vi "Setup 4 Oscilloscope.vi"() -> ()   [LabVIEW 2017]
uses:
  SignalConversion/DAQChannelRawData.ctl
  SignalConversion/ScaledData.ctl
  SignalConversion/Measrured TrapXYZ.ctl
  SignalConversion/Data Before Angle Compensation.ctl
  SignalConversion/Angle compensated data.ctl
  SignalConversion/XYZ Signals.ctl
  SignalConversion/Set TrapXYZ.ctl
  Initialization/New Param_170907.ctl
  Initialization/ManualCtrl.ctl
  Initialization/CylinderCalibrNew.ctl
  SignalConversion/DAQChannelOffsets.ctl
  <vilib>/Analysis/Matrix/Datatypes/RealMatrix.ctl
  <vilib>/Platform/TimedLoop/XDataNode/timing_clust.ctl
  <vilib>/Platform/TimedLoop/XDataNode/nitl_modes.ctl
  <vilib>/Platform/TimedLoop/XDataNode/wakeup.ctl
  <vilib>/Analysis/baseanly.llb/Mean (DBL).vi
  <vilib>/Utility/file.llb/Read Delimited Spreadsheet (DBL).vi
  <vilib>/Utility/file.llb/Write Delimited Spreadsheet (DBL).vi
  <vilib>/platform/TimedLoop/XDataNode/XDataNode.xnode
  Data aquisition/Data aquisition.lvlib
  BasicVIs/BasicVIs.lvlib
  SignalConversion/SignalConverson.lvlib
  <vilib>/Analysis/NI_AALBase.lvlib
  Initialization/FileManagement/FileManagement.lvlib
  <vilib>/Platform/TimedLoop/XDataNode/XDNodeRunTimeDep.lvlib
  Initialization/Initialization.lvlib
  <vilib>/Analysis/Matrix/NI_Matrix.lvlib
panel:
  out "Temperature":string
  out "#Recoreded":i32
  out "Frames":i32
  in  "Oscilloscope sampling Rate":i32=100
  in  "Tab Control":T1(tab)
  out "Temperature":dbl(graph)
  out "Trap height 2":dbl(graph)
  in  "Ignore HF and XYFTC calibration":bool=TRUE
  out "scan backlog:":u32
  out "no error?":bool=TRUE
  out "Torque [pNnm]":dbl(graph)
  out "Trap height":dbl(graph)
  out "Zforce [pN]":dbl(graph)
  out "ellipiticity out":dbl(knob)=10.0 scale=-0.5..0.5
  out "Vy\n            [V]":dbl(knob)=10.0 scale=-0.5..0.5
  out "Vx\n            [V]":dbl(knob)=10.0 scale=-0.5..0.5
  out "Vsum\n            [V]":dbl(knob)=10.0 scale=0.0..10.0
  out "Power meter\n            [mW]":dbl(knob)=500.0 scale=0.0..200.0
  in  "Initialize":bool
  in  "STOP":bool
  in  "Oscilloscope calibration file save path":path=path "V:/Oslo/Setup 4 temp files/Oscilloscope_offset_gain.ini.txt"
  in  "Cal 1":bool
  in  "Cal 2":bool
  in  "Temp file for calibration (channel voltages from control software)":path=path "V:/Oslo/Setup 4 temp files/all channel signals.txt"
  in  "Params measured by control program":path=path "Y:/Setup4/Setup 4 temp files/config of last run.bin"
  in  "Channel gain and offset file (mapping voltages from \"oscilloscope comuputer\" to \"control computer\")":path=path "Y:/Setup4/Setup 4 temp files/Oscilloscope_offset_gain.ini.txt"
  in  "window smooth size (default = 10 points)":i32=10
  in  "Data process in oscilloscope (2,default)":i32(ring)=2 items=["0. Do not compensate, do not calculate polarization angle", "1. Calculate angle, but do not compensate any signal", "2. Compensate all signals by angular gain", "3. Do not scale (show raw voltage signals)"]
  out "point 1 calibration":dbl[][](array[numeric])
  out "Array":T2[](array[typedef])
  out "gains and offsets of all channels":dbl[][](array[numeric])
  in  "Record all channel":bool
  out "error out":errorcluster
  out "Params out":T3={"Manual Control"={"Rotation Control"={"Phase"=0.0, "A amp (0-120)"=75.0, "B amp (0-120)"=53.3, "mean freq  [MHz]\ndefault 39.99"=40.0, "freq difference [Hz]"=2.0, "Enable A"=TRUE, "Enable B"=TRUE}, "X piezo\n [nm]"=nan, "Y peizo\n [nm]"=nan, "-Z piezo\n [nm]"=nan, "AOM0 \nPower"=nan}, "Piezo Calibr"={"Px2Vx(AO)"=nan, "Py2Vy(AO)"=nan, "Pz2Vz(AO)"=nan, "Min Px"=nan, "Min Py"=0.0, "Min Pz"=nan, "Max Px"=nan, "Max Py"=nan, "Max Pz"=nan, "Vx0 (V)"=nan, "Vy0 (V)"=nan, "Vz0 (V)"=nan}, "Instrument Calibr"={"Angular compensation coeffs"=[], "TetherCenter"={"TrapX_AO 0 [nm]"=nan, "TrapY_AO 0 [nm]"=nan, "TrapZ_AO 0 [nm]"=nan}, "XYZsignal baseline"={"Xsignal0"=nan, "Ysignal0"=nan, "Zsignal0"=nan, "Zsig slope"=nan, "Z bead0"=nan}, "S and P to Vs0"={"Vs0/P"=1.0, "Vs0/S"=1.0}, "Psi"=nan, "ePS:eRL drift correlation"={"Interc P"=nan, "Slope P"=nan, "Interc S"=nan, "Slope S"=nan}, "Current piezo volt AO"={"Vpx_AO [V]"=nan, "Vpy_AO [V]"=nan, "Vpz_AO [V]"=nan}}, "Cylinder Calibr"={"ZStiff"=nan, "Zsens"=nan, "AngStiff"=nan, "XStiff"=nan, "Xsens"=nan, "MaxEllip"=nan, "YStiff"=nan, "Ysens"=nan, "FocalShift"=nan, "Sfz"=nan, "1/Sz"=nan, "Stau"=nan, "Sfx"=nan, "1/Sx"=nan, "1/Sang"=nan, "Sfy"=nan, "1/Sy"=nan, "1/focal"=nan}, "DAQParams"={"Buffer size"=0.0, "Scanning rate"=0.0, "Average"=0.0, "Sampling rate"=0.0, "set dt"=0.0}, "DAQ channel offsets"={"A0 [V]"=0.0, "D0 [V]"=0.0, "P0  [V]"=0.0, "S0 [V]"=0.0, "L0 [V]"=0.0, "R0 [V]"=0.0, "Vpx0 [V]"=0.0, "Vpy0 [V]"=0.0, "Vpz0 [V]"=0.0, "Vsum0 [V]"=0.0, "Vpx_AO0 [V]"=0.0, "Vpy_AO0 [V]"=0.0, "Vpz_AO0 [V]"=0.0}, "Z bead polynomial coeffs"=[nan, nan, nan, nan], "Skip button ref"=refnum, "z bead lookup table"={"z signal"=[], "z bead"=[]}, "SP->power Matrix"=[], "Ms2p"=[], "Mp2s"=[], "Polynomial coeff V_px,y,z 2 position (nm)"=[], "task in"=""} {"Instrument Calibr"."Psi" format="%#_2f"; "Manual Control"."Y peizo\n [nm]" scale=0.0..7000.0; "Manual Control"."AOM0 \nPower" scale=0.0..1.0; "Manual Control"."X piezo\n [nm]" scale=0.0..7000.0; "Manual Control"."Rotation Control"."freq difference [Hz]" step=0.5; "Manual Control"."Rotation Control"."mean freq  [MHz]\ndefault 39.99" min=0.0 step=0.01; "Manual Control"."Rotation Control"."B amp (0-120)" min=0.0 max=120.0 step=0.1; "Manual Control"."Rotation Control"."A amp (0-120)" min=0.0 max=120.0 step=0.1; "Manual Control"."Rotation Control"."Phase" scale=0.0..360.0; "Manual Control"."-Z piezo\n [nm]" scale=1000.0..7000.0}
  out "Scaled data":T8
  out "all channels":dbl[][](graph)
  # "Set piezo xy and trap height to zero, turn off AOM A and B, click on \"Setup 4 Control Software: Tools: record all channel raw voltages\""
  # "Set piezo xy and trap height to max, turn on AOM A and B, set  the laser power to max and adjust the phase to achieve A detector voltage = D detector voltage (the 2nd waveform chart, show \"A and D detector [V]\"). Then click on \"Setup 4 Control Software\": tab\" Calibration Tools\" : Bottom \"record all channel raw voltages\""
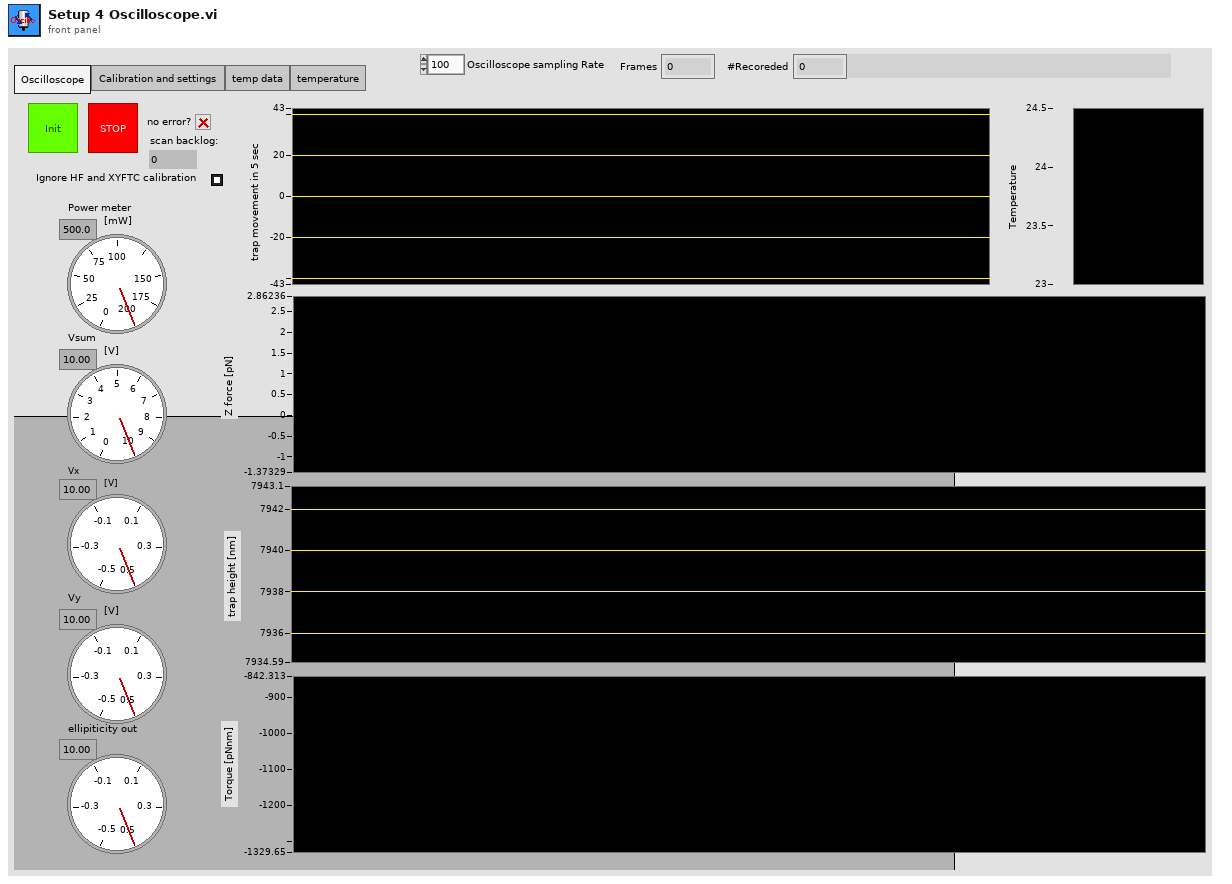
[diagram p1: front panel]
types:
  T1 = enum32{"Oscilloscope", "Calibration and settings ", "temp data", "temperature"}
  T2 = typedef "SignalConverson.lvlib/DAQChannelRawData.ctl" = cluster{"V_A' [V]":dbl, "V_D' [V]":dbl, "V_P'  [V]":dbl, "V_S' [V]":dbl, "V_L' [V]":dbl, "V_R' [V]":dbl, "V_sum' [V]":dbl, "V_x [V]":dbl, "V_y [V]":dbl, "V_px' [V]":dbl, "V_py' [V]":dbl, "V_pz' [V]":dbl, "dt [s]":dbl, "Vpx_AO [V]":dbl, "Vpy_AO [V]":dbl, "Vpz_AO [V]":dbl, "scan backlog":u32, "Counter":u32, "V_T":dbl}
  T3 = typedef "Initialization.lvlib/New Param_170907.ctl" = cluster{"Manual Control":T4, "Piezo Calibr":cluster{"Px2Vx(AO)":dbl, "Py2Vy(AO)":dbl, "Pz2Vz(AO)":dbl, "Min Px":dbl, "Min Py":dbl, "Min Pz":dbl, "Max Px":dbl, "Max Py":dbl, "Max Pz":dbl, "Vx0 (V)":dbl, "Vy0 (V)":dbl, "Vz0 (V)":dbl}, "Instrument Calibr":cluster{"Angular compensation coeffs":dbl[][], "TetherCenter":cluster{"TrapX_AO 0 [nm]":dbl, "TrapY_AO 0 [nm]":dbl, "TrapZ_AO 0 [nm]":dbl}, "XYZsignal baseline":cluster{"Xsignal0":dbl, "Ysignal0":dbl, "Zsignal0":dbl, "Zsig slope":dbl, "Z bead0":dbl}, "S and P to Vs0":cluster{"Vs0/P":dbl, "Vs0/S":dbl}, "Psi":dbl, "ePS:eRL drift correlation":cluster{"Interc P":dbl, "Slope P":dbl, "Interc S":dbl, "Slope S":dbl}, "Current piezo volt AO":cluster{"Vpx_AO [V]":dbl, "Vpy_AO [V]":dbl, "Vpz_AO [V]":dbl}}, "Cylinder Calibr":T5, "DAQParams":cluster{"Buffer size":dbl, "Scanning rate":dbl, "Average":dbl, "Sampling rate":dbl, "set dt":dbl}, "DAQ channel offsets":T6, "Z bead polynomial coeffs":dbl[], "Skip button ref":refnum<vi>, "z bead lookup table":cluster{"z signal":dbl[], "z bead":dbl[]}, "SP->power Matrix":T7, "Ms2p":T7, "Mp2s":T7, "Polynomial coeff V_px,y,z 2 position (nm)":dbl[][], "task in":refnum<k21>}
  T4 = typedef "Initialization.lvlib/ManualCtrl.ctl" = cluster{"Rotation Control":cluster{"Phase":dbl, "A amp (0-120)":dbl, "B amp (0-120)":dbl, "mean freq  [MHz]\ndefault 39.99":dbl, "freq difference [Hz]":dbl, "Enable A":bool, "Enable B":bool}, "X piezo\n [nm]":dbl, "Y peizo\n [nm]":dbl, "-Z piezo\n [nm]":dbl, "AOM0 \nPower":dbl}
  T5 = typedef "Initialization.lvlib/CylinderCalibrNew.ctl" = cluster{"ZStiff":dbl, "Zsens":dbl, "AngStiff":dbl, "XStiff":dbl, "Xsens":dbl, "MaxEllip":dbl, "YStiff":dbl, "Ysens":dbl, "FocalShift":dbl, "Sfz":dbl, "1/Sz":dbl, "Stau":dbl, "Sfx":dbl, "1/Sx":dbl, "1/Sang":dbl, "Sfy":dbl, "1/Sy":dbl, "1/focal":dbl}
  T6 = typedef "SignalConverson.lvlib/DAQChannelOffsets.ctl" = cluster{"A0 [V]":dbl, "D0 [V]":dbl, "P0  [V]":dbl, "S0 [V]":dbl, "L0 [V]":dbl, "R0 [V]":dbl, "Vpx0 [V]":dbl, "Vpy0 [V]":dbl, "Vpz0 [V]":dbl, "Vsum0 [V]":dbl, "Vpx_AO0 [V]":dbl, "Vpy_AO0 [V]":dbl, "Vpz_AO0 [V]":dbl}
  T7 = typedef "NI_Matrix.lvlib/RealMatrix.ctl" = dbl[][]
  T8 = typedef "SignalConverson.lvlib/ScaledData.ctl" = cluster{"Measured TrapXYZ":T9, "Data before TCT":T10, "Data after angle compensation":T11, "X,Y,Z signal":T12, "Set TrapXYZ":T13}
  T9 = typedef "SignalConverson.lvlib/Measrured TrapXYZ.ctl" = cluster{"TrapX [nm]":dbl, "TrapY [nm]":dbl, "TrapZ [nm]":dbl}
  T10 = typedef "SignalConverson.lvlib/Data Before Angle Compensation.ctl" = cluster{"V_A [V]":dbl, "V_D [V]":dbl, "V_P [V]":dbl, "V_S [V]":dbl, "V_L [V]":dbl, "V_R [V]":dbl, "V_sum [V]":dbl, "V_x [V]":dbl, "V_y [V]":dbl, "P power [mW]":dbl, "S power [mW]":dbl}
  T11 = typedef "SignalConverson.lvlib/Angle compensated data.ctl" = cluster{"angle compensated P power [W]":dbl, "angle compensated S power [W]":dbl, "angle compensated V_L":dbl, "angle compensated V_R":dbl, "angle compensated V_sum [V]":dbl, "angle compensated V_x [V]":dbl, "angle compensated V_y [V]":dbl, "Psi [rad]":dbl, "Laser power before objective[W]":dbl, "E_in":dbl, "E_out":dbl, "Delta E":dbl}
  T12 = typedef "SignalConverson.lvlib/XYZ Signals.ctl" = cluster{"X signal":dbl, "Y signal":dbl, "Z signal":dbl}
  T13 = typedef "SignalConverson.lvlib/Set TrapXYZ.ctl" = cluster{"TrapX (AO) [nm]":dbl, "TrapY (AO) [nm]":dbl, "TrapZ (AO) [nm]":dbl}
  T14 = typedef "XDNodeRunTimeDep.lvlib/timing_clust.ctl" = cluster{"Expected End [f-1]":u64, "Actual End [f-1]":u64, "Finished Late? [f-1]":bool, "Expected End [i-1]":u64, "Actual End [i-1]":u64, "Finished Late? [i-1]":bool, "Expected Start [i]":u64, "Actual Start [i]":u64, "Expected Start [f]":u64, "Actual Start [f]":u64, "Source Name":string, "Structure Name":string, "Period":i64, "Deadline":i64, "Offset":i64, "Start":i64, "Priority":i32, "Timeout":i32, "Mode":T15, "Wakeup Reason":T16, "Error":errorcluster, "Source Type":string, "Secondary Source Type":string, "Global End Time":u64, "Global Start Time":u64, "Frame Duration":u64, "Iteration Duration":u64, "Assigned CPU":i32, "I/O Scan Engine Mode":u32}
  T15 = typedef "XDNodeRunTimeDep.lvlib/nitl_modes.ctl" = enum32{"No Change", "Process missed periods, maintain original phase", "Discard missed periods, maintain original phase", "Process missed periods, ignore original phase", "Discard missed periods, ignore original phase"}
  T16 = typedef "XDNodeRunTimeDep.lvlib/wakeup.ctl" = enum32{"Normal", "Aborted", "Asynchronous wakeup", "Timing source error", "Timed loop error", "Timeout"}
  T17 = typedef "SignalConverson.lvlib/Physical Quantitites.ctl" = cluster{"Fz [pN]":dbl, "Zext [nm]":dbl, "Tau [pNnm]":dbl, "Turn":dbl, "Fx [pN]":dbl, "Xext [nm]":dbl, "Fy [pN]":dbl, "Yext [nm]":dbl, "time [s]":dbl, "Delta Z signal":dbl, "Delta Z bead [nm]":dbl, "Z bead [nm]":dbl, "Delta TrapZ [nm]":dbl, "Delta Xsignal":dbl, "X bead [nm]":dbl, "Delta Ysignal":dbl, "Y bead [nm]":dbl, "Stop Condition":dbl}
  T18 = enum16{"open", "replace", "create", "open or create", "replace or create", "replace or create with confirmation"}
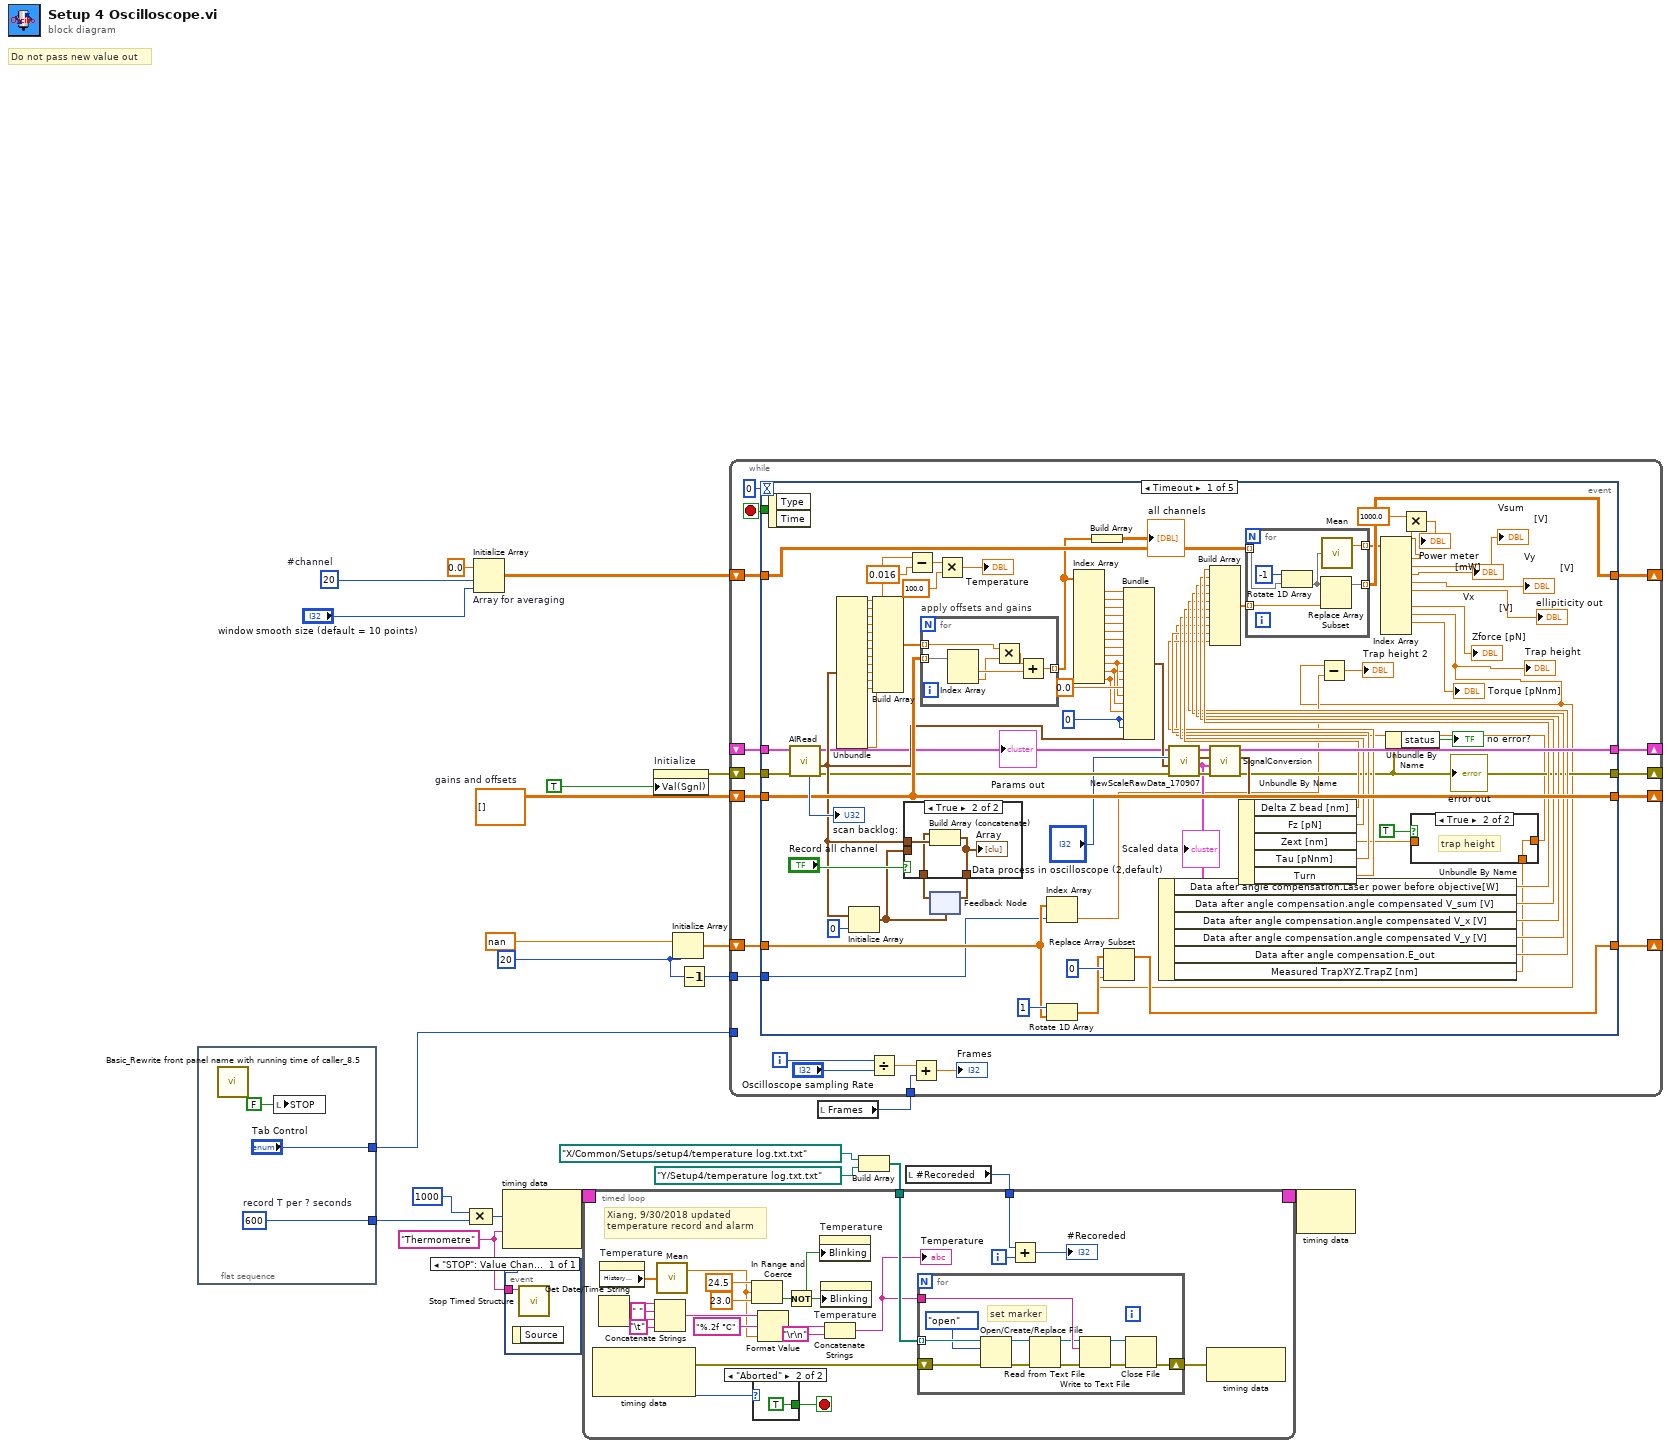
[diagram p0: block diagram]
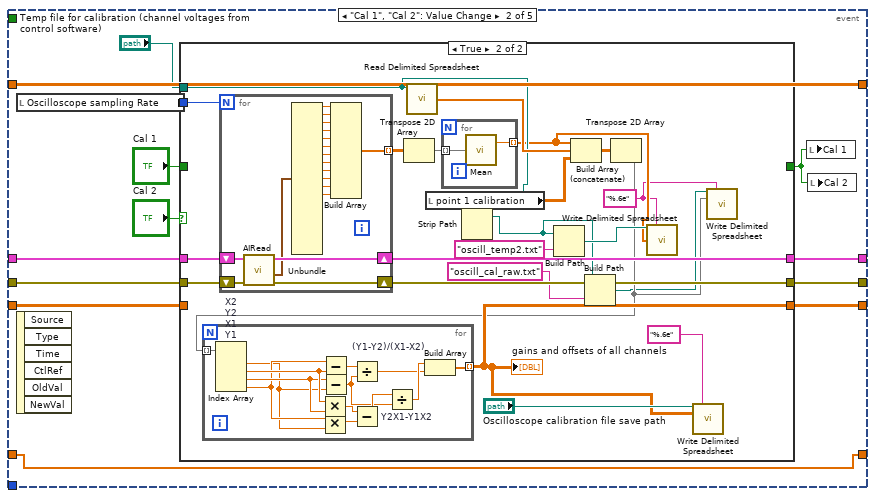
[diagram p5: hidden frame]
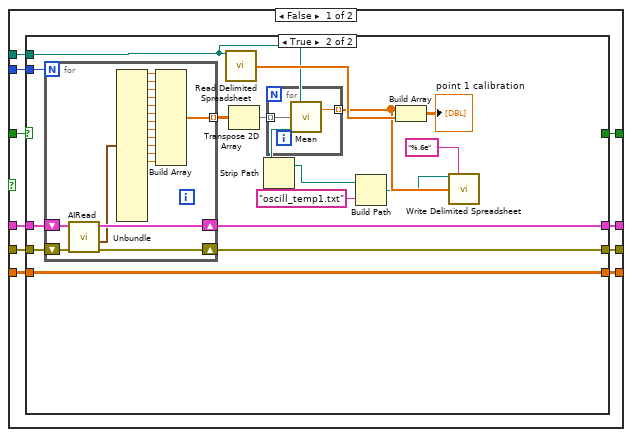
[diagram p6: hidden frame]
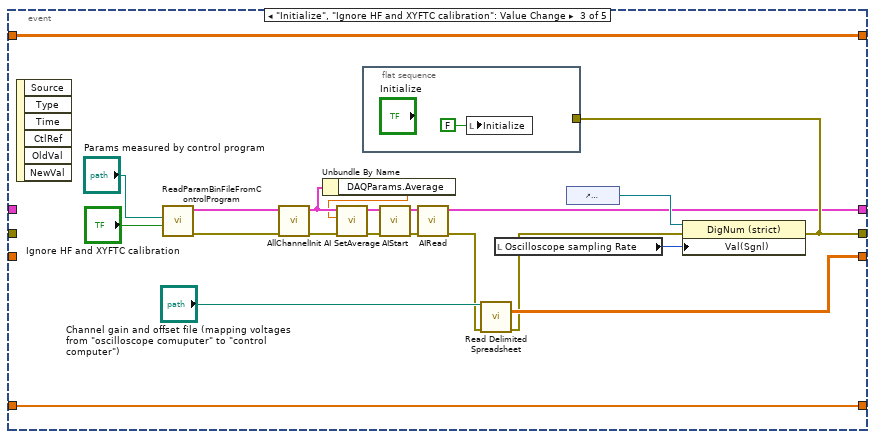
[diagram p8: hidden frame]
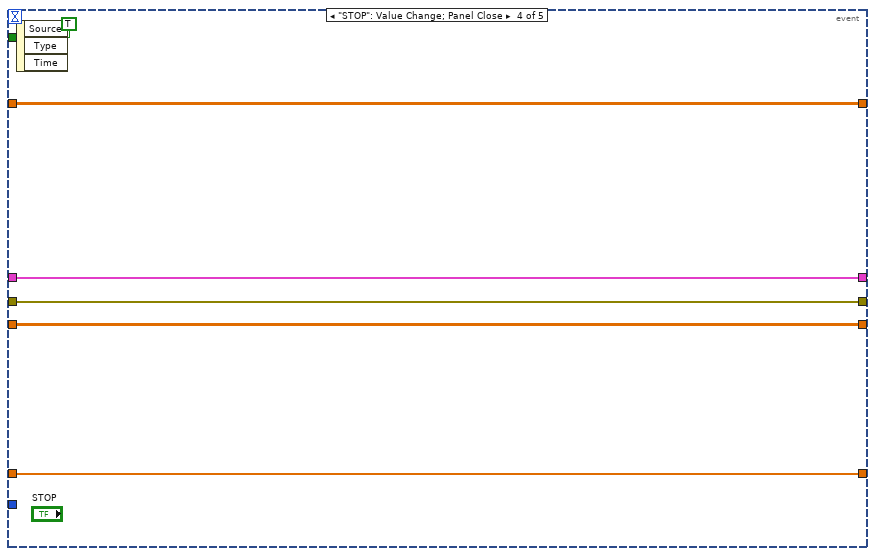
[diagram p9: hidden frame]
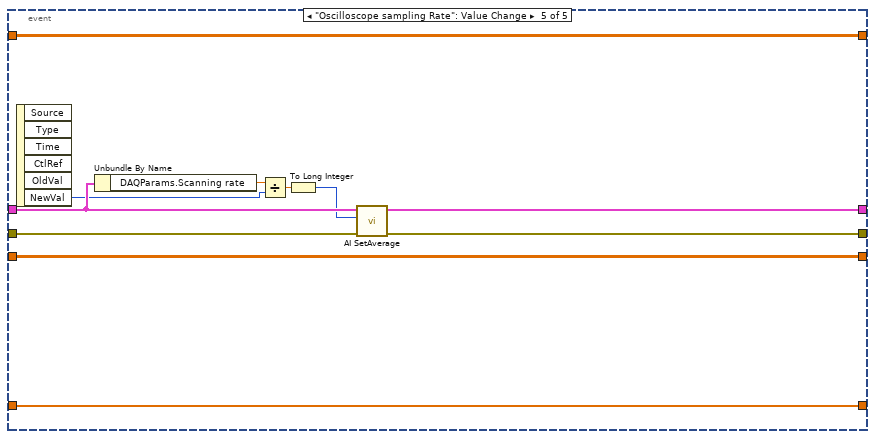
[diagram p10: hidden frame]
diagram:
  w7 = "Thermometre" ("Structure Name")
  w15 = 20 ("dimension size")
  w17 = 20  # #channel
  w19 = dbl[][] []  # gains and offsets
  # "Do not pass new value out"
  n1 = flat-sequence {
    tunnel: [w25] -> w5
    tunnel: ["Tab Control"] -> w4
    frame #0 {
      w25 = 600  # record T per ? seconds
      n2 = call "Basic_Rewrite front panel name with running time of caller_8.5.vi"() -> ()  [unwired: 12 in]
      n3 = local write "STOP"(FALSE ("STOP")) -> ()
    }
  }
  n4 = Compound Arithmetic op=MULTIPLY(i64 1000 ("Period"), w5) -> (w6:i64)
  n5 = Initialize Array "Array for averaging"(0.0 ("element"), w17, "window smooth size (default = 10 points)") -> (w20:dbl[][])
  n6 = node-c288(w6, w7) -> (w13:T14)
  n7 = event shown="[0] \"STOP\": Value Change" {
    selector: _ -> [_]
    dyn-events: _ -> [_]
    timeout: _ -> [_]
    tunnel: w7 -> [w27]
    event "STOP": Value Change {
      n8 = event-data() -> ()  [unwired: 1 in, 1 out]
      n9 = call <vilib>:"Stop Timed Structure.vi"("name"=w27) -> ()  [unwired: 10 in, 1 out]
    }
  }
  n10 = property on="Initialize" class="Bool (strict)"("Val(Sgnl)"=TRUE ("Value (Signaling)")) -> (error out=w23:errorcluster)  [unwired: 2 in, 1 out]
  n11 = Initialize Array(nan ("element"), w15) -> (w16:dbl[])
  n12 = Decrement(x=w15) -> (x-1=w14:i32)
  n13 = local read "Frames"() -> (w1:i32)
  n14 = while {
    shift-right: [w44] -> _
    shift-left: w23 -> [w45]
    shift-right: [w43] -> _
    shift-left: _ -> [w41]
    shift-right: [w39] -> _
    shift-left: w19 -> [w38]
    shift-right: [w36] -> _
    shift-left: w20 -> [w37]
    shift-right: [w32] -> _
    shift-left: w16 -> [w33]
    tunnel: w14 -> [w31]
    tunnel: w4 -> [_]
    tunnel: w1 -> [w30]
    i -> [w35]
    stop <- w40 stop-if-true
    n15 = event shown="[0] Timeout" {
      selector: _ -> [_ _ _ _ _]
      dyn-events: _ -> [_ _ _ _ _]
      timeout: 0 -> [_ _ _ _ _]
      tunnel: w41 -> [w122 w157 _ w300 w308]
      tunnel: w45 -> [w135 w156 _ w295 w311]
      tunnel: [w71 w159 w284 w295 w310] -> w44
      tunnel: [w96 w158 w277 w300 w309] -> w43
      tunnel: [_ _ _ TRUE ("Value (Signaling)") _] -> w40
      tunnel: [w115 w160 w281 w298 w304] -> w39
      tunnel: w38 -> [w115 w161 _ w298 w304]
      tunnel: w37 -> [w80 w167 w283 w297 w303]
      tunnel: [w79 w167 w283 w297 w303] -> w36
      tunnel: w33 -> [w55 w155 w273 w296 w301]
      tunnel: [w56 w155 w273 w296 w301] -> w32
      tunnel: w31 -> [w51 _ _ _ _]
      event Timeout {
        w100 = u32 0 ("scan backlog")
        n16 = event-data() -> ()  [unwired: 1 in, 2 out]
        n17 = call "AIRead.vi"("error in (no error)"=w135, "Params in"=w122) -> ("error out"=w99:errorcluster, "All Channel Names"=w114:T2, "Params out"=w67:T3, "scan backlog"=→"scan backlog:":u32)  [unwired: 5 in, 1 out]
        "Params out" <- w67
        n18 = Unbundle(w114) -> ("V_A' [V]"=w134:dbl, "V_D' [V]"=w133:dbl, "V_P'  [V]"=w132:dbl, "V_S' [V]"=w131:dbl, "V_L' [V]"=w130:dbl, "V_R' [V]"=w129:dbl, "V_sum' [V]"=w128:dbl, "V_x [V]"=w127:dbl, "V_y [V]"=w126:dbl, "V_px' [V]"=w125:dbl, "V_py' [V]"=w124:dbl, "V_pz' [V]"=w123:dbl, "V_T"=w47:dbl)  [unwired: 6 out]
        n19 = Initialize Array(w114, 0 ("dimension size")) -> (w117:T2[])
        n20 = Build Array(w134, w133, w132, w131, w130, w129, w128, w127, w126, w125, w124, w123) -> (w116:dbl[])
        n21 = Subtract(x=w47, y=0.016) -> (x-y=w48:dbl)
        n22 = for "apply offsets and gains" {
          tunnel: w116 -> [w147] mode=indexing
          tunnel: w115 -> [w150] mode=indexing
          tunnel: [w145] -> w69 mode=indexing
          n23 = Index Array(array=w150) -> (element #1=w149:dbl, element #2=w148:dbl)  [unwired: 2 in]
          n24 = Multiply(x=w147, y=w148) -> (x*y=w146:dbl)
          n25 = Add(x=w146, y=w149) -> (x+y=w145:dbl)
        }
        n26 = feedback #1(w117) -> (w118:T2[])
        n27 = case shown="True" "Record all channel" {
          tunnel: w114 -> [_ w154]
          tunnel: [w151 w152] -> w119
          tunnel: w118 -> [_ w153]
          tunnel: w117 -> [w151 _]
          frame False {
          }
          frame True {
            n28 = Build Array (concatenate)(w153, w154) -> (w152:T2[])
            "Array" <- w152
          }
        }
        n29 = feedback-in #1(w119) -> ()
        n30 = Multiply(x=w48, y=100.0) -> (x*y=→"Temperature":dbl)
        n31 = Index Array(array=w55, index=w51) -> (element=w54:dbl)
        n32 = Rotate 1D Array(1:w55, 2:1 ("n")) -> (0:w57:dbl[])
        n33 = Index Array(array=w69) -> (element #1=w113:dbl, element #2=w111:dbl, element #3=w112:dbl, element #4=w110:dbl, element #5=w109:dbl, element #6=w108:dbl, element #7=w107:dbl, element #8=w104:dbl, element #9=w106:dbl, element #10=w103:dbl, element #11=w102:dbl, element #12=w101:dbl)  [unwired: 12 in]
        n34 = Build Array(w69) -> (→"all channels":dbl[][])
        n35 = Bundle(cluster=w114, "V_A' [V]"=w113, "V_D' [V]"=w111, "V_P'  [V]"=w112, "V_S' [V]"=w110, "V_L' [V]"=w109, "V_R' [V]"=w108, "V_sum' [V]"=w107, "V_x [V]"=w104, "V_y [V]"=w106, "V_px' [V]"=w103, "V_py' [V]"=w102, "V_pz' [V]"=w101, "dt [s]"=0.0, "Vpx_AO [V]"=w103, "Vpy_AO [V]"=w102, "Vpz_AO [V]"=w101, "scan backlog"=w100, "Counter"=w100) -> (w91:T2)  [unwired: 1 in]
        n36 = call "NewScaleRawData_170907.vi"("error in (no error)"=w99, "All DAQ channels"=w91, "Scale Option"="Data process in oscilloscope (2,default)", "Params in"=w67) -> ("error out"=w98:errorcluster, "Scaled data"=w92:T8, "All DAQ channels out"=w94:T2, "Params out"=w97:T3)  [unwired: 1 in]
        "Scaled data" <- w92
        n37 = Unbundle By Name(w92) -> ("Data after angle compensation.Laser power before objective[W]"=w90:dbl, "Data after angle compensation.angle compensated V_sum [V]"=w89:dbl, "Data after angle compensation.angle compensated V_x [V]"=w88:dbl, "Data after angle compensation.angle compensated V_y [V]"=w87:dbl, "Data after angle compensation.E_out"=w86:dbl, "Measured TrapXYZ.TrapZ [nm]"=w63:dbl)
        n38 = call "SignalConversion.vi"("error in (no error)"=w98, "All data after scaling"=w92, "All DAQ channels"=w94, "Params in"=w97) -> ("error out"=w71:errorcluster, "Physical Quantities cluster out"=w93:T17, "Params out"=w96:T3)  [unwired: 5 in]
        "error out" <- w71
        n39 = Unbundle By Name(w93) -> ("Delta Z bead [nm]"=w85:dbl, "Fz [pN]"=w84:dbl, "Zext [nm]"=w62:dbl, "Tau [pNnm]"=w83:dbl, "Turn"=w82:dbl)
        n40 = Unbundle By Name(w71) -> ("status"=→"no error?":bool)
        n41 = case shown="True" TRUE {
          tunnel: w63 -> [_ w138]
          tunnel: [w137 w138] -> w61
          tunnel: w62 -> [w137 _]
          frame False {
            # "Z extension\n(too noisy)"
          }
          frame True {
            # "trap height"
          }
        }
        n42 = Build Array(w90, w89, w88, w87, w86, w85, w84, w61, w83, w82) -> (w81:dbl[])
        n43 = for {
          tunnel: w81 -> [w143] mode=indexing
          tunnel: w80 -> [w142] mode=indexing
          tunnel: [w141] -> w79 mode=indexing
          tunnel: [w139] -> w78 mode=indexing
          n44 = Rotate 1D Array(1:w142, 2:-1 ("n")) -> (0:w140:dbl[])
          n45 = Replace Array Subset(array=w140, new element=w143) -> (w141:dbl[])  [unwired: 1 in]
          n46 = call-poly <vilib>:"Mean.vi"("X"=w140) -> ("mean"=w139:dbl)  [unwired: 1 out]
        }
        n47 = Index Array(array=w78) -> (element #1=w65:dbl, element #2=→"Vsum\n            [V]":dbl, element #3=→"Vx\n            [V]":dbl, element #4=→"Vy\n            [V]":dbl, element #5=→"ellipiticity out":dbl, element #7=→"Zforce [pN]":dbl, element #8=w53:dbl, element #9=→"Torque [pNnm]":dbl)  [unwired: 10 in, 2 out]
        "Trap height" <- w53
        n48 = Replace Array Subset(array=w57, new element=w53, index=0) -> (w56:dbl[])
        n49 = Subtract(x=w53, y=w54) -> (x-y=→"Trap height 2":dbl)
        n50 = Multiply(x=1000.0, y=w65) -> (x*y=→"Power meter\n            [mW]":dbl)
      }
      event "Cal 1", "Cal 2": Value Change {
        n51 = local read "Oscilloscope sampling Rate"() -> (w163:i32)
        n52 = event-data() -> ()  [unwired: 1 in, 6 out]
        n53 = case shown="True" "Cal 2" {
          tunnel: "Cal 1" -> [w177 _]
          tunnel: w163 -> [w176 w231]
          tunnel: [w175 w229] -> w160
          tunnel: [w174 w237] -> w158
          tunnel: [w173 w236] -> w159
          tunnel: w157 -> [w172 w234]
          tunnel: w156 -> [w171 w235]
          tunnel: w161 -> [w170 _]
          tunnel: "Temp file for calibration (channel voltages from control software)" -> [w169 w224]
          tunnel: [w168 _] -> w166
          frame False {
            n54 = case shown="True" w177 {
              selector: w177 -> [w178 _]
              tunnel: w172 -> [w181 w197]
              tunnel: w171 -> [w180 w196]
              tunnel: [w181 w194] -> w174
              tunnel: [w180 w195] -> w173
              tunnel: [w179 w190] -> w175
              tunnel: w170 -> [w179 w190]
              tunnel: w176 -> [_ w192]
              tunnel: w169 -> [_ w185]
              tunnel: [w178 _] -> w168
              frame False {
              }
              frame True {
                n55 = for {
                  N: w192 -> [_]
                  shift-right: [w215] -> w194
                  shift-left: w197 -> [w217]
                  shift-right: [w214] -> w195
                  shift-left: w196 -> [w216]
                  tunnel: [w200] -> w191 mode=indexing
                  n56 = call "AIRead.vi"("error in (no error)"=w216, "Params in"=w217) -> ("error out"=w214:errorcluster, "All Channel Names"=w213:T2, "Params out"=w215:T3)  [unwired: 5 in, 2 out]
                  n57 = Unbundle(w213) -> ("V_A' [V]"=w212:dbl, "V_D' [V]"=w211:dbl, "V_P'  [V]"=w210:dbl, "V_S' [V]"=w209:dbl, "V_L' [V]"=w208:dbl, "V_R' [V]"=w207:dbl, "V_sum' [V]"=w206:dbl, "V_x [V]"=w205:dbl, "V_y [V]"=w204:dbl, "V_px' [V]"=w203:dbl, "V_py' [V]"=w202:dbl, "V_pz' [V]"=w201:dbl)  [unwired: 7 out]
                  n58 = Build Array(w212, w211, w210, w209, w208, w207, w206, w205, w204, w203, w202, w201) -> (w200:dbl[])
                }
                n59 = call-poly <vilib>:"Read Delimited Spreadsheet.vi"("file path (dialog if empty)"=w185) -> ("first row"=w188:dbl[])  [unwired: 9 in, 5 out]
                n60 = Transpose 2D Array(2D array=w191) -> (transposed array=w193:dbl[][])
                n61 = Strip Path(path=w185) -> (stripped path=w186:path)  [unwired: 1 out]
                n62 = for {
                  tunnel: w193 -> [w199] mode=indexing
                  tunnel: [w198] -> w184 mode=indexing
                  n63 = call-poly <vilib>:"Mean.vi"("X"=w199) -> ("mean"=w198:dbl)  [unwired: 1 out]
                }
                n64 = Build Path(base path=w186, name or relative path="oscill_temp1.txt") -> (appended path=w183:path)
                n65 = Build Array(w184, w188) -> (→"point 1 calibration":dbl[][])
                n66 = call-poly <vilib>:"Write Delimited Spreadsheet.vi"("file path (dialog if empty)"=w183, "format (%.3f)"="%.6e", "1D data"=w184) -> ()  [unwired: 11 in, 2 out]
              }
            }
          }
          frame True {
            w218 = "%.6e" ("format (%.3f)")
            n67 = for {
              N: w231 -> [_]
              shift-right: [w270] -> w237
              shift-left: w234 -> [w272]
              shift-right: [w269] -> w236
              shift-left: w235 -> [w271]
              tunnel: [w255] -> w238 mode=indexing
              n68 = call "AIRead.vi"("error in (no error)"=w271, "Params in"=w272) -> ("error out"=w269:errorcluster, "All Channel Names"=w268:T2, "Params out"=w270:T3)  [unwired: 5 in, 2 out]
              n69 = Unbundle(w268) -> ("V_A' [V]"=w267:dbl, "V_D' [V]"=w266:dbl, "V_P'  [V]"=w265:dbl, "V_S' [V]"=w264:dbl, "V_L' [V]"=w263:dbl, "V_R' [V]"=w262:dbl, "V_sum' [V]"=w261:dbl, "V_x [V]"=w260:dbl, "V_y [V]"=w259:dbl, "V_px' [V]"=w258:dbl, "V_py' [V]"=w257:dbl, "V_pz' [V]"=w256:dbl)  [unwired: 7 out]
              n70 = Build Array(w267, w266, w265, w264, w263, w262, w261, w260, w259, w258, w257, w256) -> (w255:dbl[])
            }
            n71 = Transpose 2D Array(2D array=w238) -> (transposed array=w239:dbl[][])
            n72 = call-poly <vilib>:"Read Delimited Spreadsheet.vi"("file path (dialog if empty)"=w224) -> ("first row"=w227:dbl[])  [unwired: 9 in, 5 out]
            n73 = local read "point 1 calibration"() -> (w233:dbl[][])
            n74 = for {
              tunnel: w239 -> [w254] mode=indexing
              tunnel: [w253] -> w223 mode=indexing
              n75 = call-poly <vilib>:"Mean.vi"("X"=w254) -> ("mean"=w253:dbl)  [unwired: 1 out]
            }
            n76 = Strip Path(path=w224) -> (stripped path=w220:path)  [unwired: 1 out]
            n77 = Build Path(base path=w220, name or relative path="oscill_temp2.txt") -> (appended path=w225:path)
            n78 = Build Array (concatenate)(w223, w227, w233) -> (w232:dbl[][])
            n79 = Build Path(base path=w220, name or relative path="oscill_cal_raw.txt") -> (appended path=w219:path)
            n80 = Transpose 2D Array(2D array=w232) -> (transposed array=w222:dbl[][])
            n81 = for {
              tunnel: w222 -> [w252] mode=indexing
              tunnel: [w240] -> w229 mode=indexing
              n82 = Index Array "X2\nY2\nX1\nY1"(array=w252) -> (element #1=w247:dbl, element #2=w250:dbl, element #3=w249:dbl, element #4=w248:dbl)  [unwired: 4 in]
              n83 = Multiply(x=w250, y=w249) -> (x*y=w246:dbl)
              n84 = Multiply(x=w248, y=w247) -> (x*y=w245:dbl)
              n85 = Subtract(x=w248, y=w250) -> (x-y=w251:dbl)
              n86 = Subtract(x=w249, y=w247) -> (x-y=w243:dbl)
              n87 = Divide "(Y1-Y2)/(X1-X2)"(x=w251, y=w243) -> (x/y=w241:dbl)
              n88 = Subtract "Y2X1-Y1X2"(x=w246, y=w245) -> (x-y=w244:dbl)
              n89 = Divide(x=w244, y=w243) -> (x/y=w242:dbl)
              n90 = Build Array(w242, w241) -> (w240:dbl[])
            }
            "gains and offsets of all channels" <- w229
            n91 = call-poly <vilib>:"Write Delimited Spreadsheet.vi"("file path (dialog if empty)"=w225, "format (%.3f)"=w218, "1D data"=w223) -> ()  [unwired: 11 in, 2 out]
            n92 = call-poly <vilib>:"Write Delimited Spreadsheet.vi"("file path (dialog if empty)"="Oscilloscope calibration file save path", "format (%.3f)"="%.6e", "2D data"=w229) -> ()  [unwired: 11 in, 2 out]
            n93 = call-poly <vilib>:"Write Delimited Spreadsheet.vi"("file path (dialog if empty)"=w219, "format (%.3f)"=w218, "2D data"=w222) -> ()  [unwired: 11 in, 2 out]
          }
        }
        n94 = local write "Cal 1"(w166) -> ()
        n95 = local write "Cal 2"(w166) -> ()
      }
      event "Initialize", "Ignore HF and XYFTC calibration": Value Change {
        n96 = event-data() -> ()  [unwired: 1 in, 6 out]
        n97 = call "ReadParamBinFileFromControlProgram.vi"("file path in"="Params measured by control program", "Ignore HF and XYFTC calibration"="Ignore HF and XYFTC calibration") -> ("Params out"=w276:T3, "error out"=w278:errorcluster)  [unwired: 5 in, 2 out]
        n98 = call "AllChannelInit.vi"("error in (no error)"=w278, "Input params"=w276) -> ("error out"=w290:errorcluster, "Output cluster"=w291:T3)  [unwired: 4 in]
        n99 = Unbundle By Name(w291) -> ("DAQParams.Average"=w288:dbl)
        n100 = call "AI SetAverage.vi"("error in"=w290, "Number to average"=w288, "params in"=w291) -> ("error out"=w285:errorcluster, "params out"=w289:T3)  [unwired: 3 in]
        n101 = flat-sequence {
          tunnel: w284 -> [_]
          frame #0 {
            n102 = local write "Initialize"(FALSE ("Initialize")) -> ()
          }
        }
        n103 = call "AIStart.vi"("error in (no error)"=w285, "Params in"=w289) -> ("error out"=w287:errorcluster, "Params out"=w286:T3)  [unwired: 4 in]
        n104 = call "AIRead.vi"("error in (no error)"=w287, "Params in"=w286) -> ("error out"=w280:errorcluster, "Params out"=w277:T3)  [unwired: 5 in, 3 out]
        n105 = call-poly <vilib>:"Read Delimited Spreadsheet.vi"("file path (dialog if empty)"="Channel gain and offset file (mapping voltages from \"oscilloscope comuputer\" to \"control computer\")", "error in (no error)"=w280) -> ("all rows"=w281:dbl[][], "error out"=w279:errorcluster)  [unwired: 8 in, 4 out]
        n106 = local read "Oscilloscope sampling Rate"() -> (w293:i32)
        n107 = control-ref of="Oscilloscope sampling Rate"() -> (w292:refnum<vi>)
        n108 = property on="Property Node" class="DigNum (strict)"(reference=w292, error in=w279, "Val(Sgnl)"=w293) -> (error out=w284:errorcluster)  [unwired: 1 out]
      }
      event "STOP": Value Change; Panel Close {
        n109 = event-data() -> ()  [unwired: 1 in, 3 out]
      }
      event "Oscilloscope sampling Rate": Value Change {
        n110 = event-data() -> ("NewVal"=w302:i32)  [unwired: 1 in, 5 out]
        n111 = Unbundle By Name(w308) -> ("DAQParams.Scanning rate"=w305:dbl)
        n112 = Divide(x=w305, y=w302) -> (x/y=w307:dbl)
        n113 = To Long Integer(number=w307) -> (32bit integer=w306:i32)
        n114 = call "AI SetAverage.vi"("error in"=w311, "Number to average"=w306, "params in"=w308) -> ("error out"=w310:errorcluster, "params out"=w309:T3)  [unwired: 3 in]
      }
    }
    n115 = Divide(x=w35, y="Oscilloscope sampling Rate") -> (x/y=w29:dbl)
    n116 = Add(x=w29, y=w30) -> (x+y=→"Frames":dbl)
  }
  n117 = Build Array(path "X:/Common/Setups/setup4/temperature log.txt.txt", path "Y:/Setup4/temperature log.txt.txt") -> (w8:path[])
  n118 = local read "#Recoreded"() -> (w2:i32)
  n119 = timed-loop {
    timing: w13 -> [_]
    timing-out: [_] -> w12
    tunnel: w8 -> [w328]
    tunnel: w2 -> [w312]
    i -> [w314]
    stop <- w333 stop-if-true
    # "Xiang, 9/30/2018 updated\ntemperature record and alarm"
    n120 = node-c288() -> (w318:errorcluster, w334:T16)  [unwired: 1 in]
    n121 = Get Date/Time String() -> (date string=w329:string, time string=w330:string)  [unwired: 3 in]
    n122 = property on="Temperature" class="WFChart (strict)"() -> ("History Data"=w316:dbl[])  [unwired: 2 in, 2 out]
    n123 = Concatenate Strings(w329, " " ("string"), w330, "\t") -> (w326:string)
    n124 = call-poly <vilib>:"Mean.vi"("X"=w316) -> ("mean"=w315:dbl)  [unwired: 1 out]
    n125 = In Range and Coerce(upper limit=24.5, x=w315, lower limit=23.0 ("y")) -> (In Range?=w319:bool)  [unwired: 1 out]
    n126 = case shown="\"Aborted\"" w334 {
      tunnel: [_ TRUE] -> w333
      frame "Normal", Default {
      }
      frame "Aborted" {
      }
    }
    n127 = Format Value(string ("")=w326, format string="%.2f °C", value (0)=w315) -> (output string=w324:string)
    n128 = Not(x=w319) -> (.not. x?=w317:bool)
    n129 = property on="Temperature" class="WFChart (strict)"("Blinking"=w317) -> ()  [unwired: 2 in, 2 out]
    n130 = property on="Temperature" class="Str"("Blinking"=w317) -> ()  [unwired: 2 in, 2 out]
    n131 = Concatenate Strings(w324, "\r\n") -> (w321:string)
    "Temperature" <- w321
    n132 = for {
      tunnel: w328 -> [w345] mode=indexing
      shift-right: [w341] -> w327
      shift-left: w318 -> [w342]
      tunnel: w321 -> [w339]
      # "set marker"
      n133 = Open/Create/Replace File(file path (use dialog)=w345, error in=w342, operation (0:open)=T18."open") -> (refnum out=w337:refnum<file>, error out=w338:errorcluster)  [unwired: 3 in, 1 out]
      n134 = Read from Text File(file (use dialog)=w337, error in=w338) -> (refnum out=w336:refnum<file>, error out=w335:errorcluster)  [unwired: 2 in, 2 out]
      n135 = Write to Text File(file (use dialog)=w336, text=w339, error in=w335) -> (refnum out=w343:refnum<file>, error out=w344:errorcluster)  [unwired: 1 in, 1 out]
      n136 = Close File(refnum=w343, error in=w344) -> (error out=w341:errorcluster)  [unwired: 1 out]
    }
    n137 = Add(x=w312, y=w314) -> (x+y=→"#Recoreded":i32)
    n138 = node-c288(w327) -> ()  [unwired: 1 out]
  }
  n139 = node-c288(w12) -> ()  [unwired: 1 out]
